vi "SwitchCombo.vi"() -> ()   [LabVIEW 2016]
panel:
  in  "SwitchCombo":i32[](array[numeric])
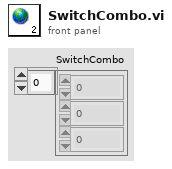
[diagram p1: front panel]
diagram:
